vi "E2_Master.vi"() -> ()   [LabVIEW 2020]
uses:
  <vilib>/Instr/_visa.llb/VISA Configure Serial Port (Instr).vi
panel:
  out "Error":errorcluster
  in  "Log":bool
  in  "UpdateTime":bool
  in  "ClearShutdown":bool
  in  "ClearWakeup":bool
  in  "Custom String":string
  in  "SendCustom":bool
  in  "ClearErrors":bool
  in  "Set Shutdown":bool
  in  "Shutdown Time":timestamp
  in  "Wakeup Time":timestamp
  in  "Set Wakeup":bool
  in  "Stop":bool
  in  "Start":bool
  in  "Write Buffer":string
  out "Laser":string
  out "Pump":string
  in  "Disconnect":bool
  in  "Initialize":bool
  in  "VISA Resource Name":refnum<visa-resource-name>
  in  "Resource Name":refnum<visa-resource-name>="Element2"
  in  "Status":bool
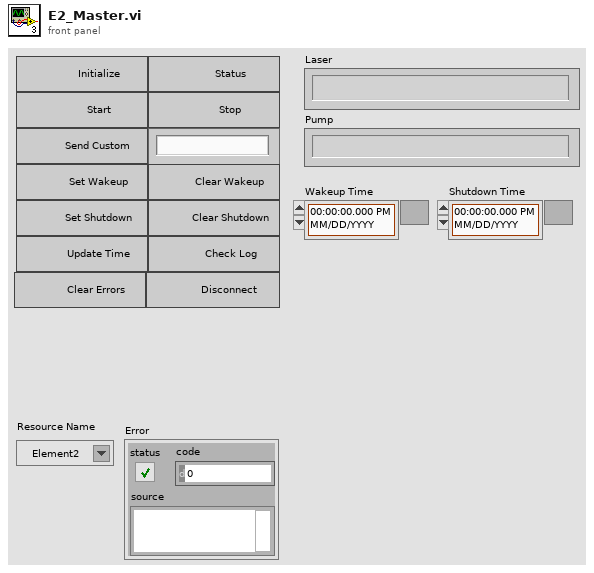
[diagram p1: front panel]
types:
  T1 = enum32{"Invalid", "Standard", "Closed", "Hidden", "Minimized", "Maximized"}
  T2 = enum32{"invalid app kind", "Development System", "Run Time System", "Student Edition", "Embedded LabVIEW", "Evaluation", "Custom"}
  T3 = enum16{"open", "replace", "create", "open or create", "replace or create", "replace or create with confirmation"}
  T4 = cluster{"Core":cluster{"Current VI Reference":refnum<vi>, "Close Panel on Exit?":bool}, "Your Boolean data":bool, "Your string data":string, "VISA Resource Name":refnum<visa-resource-name>, "Write Buffer":string, "Laser Status":string, "Pump Status":string}
  T5 = cluster{"Current VI Reference":refnum<vi>, "Close Panel on Exit?":bool}
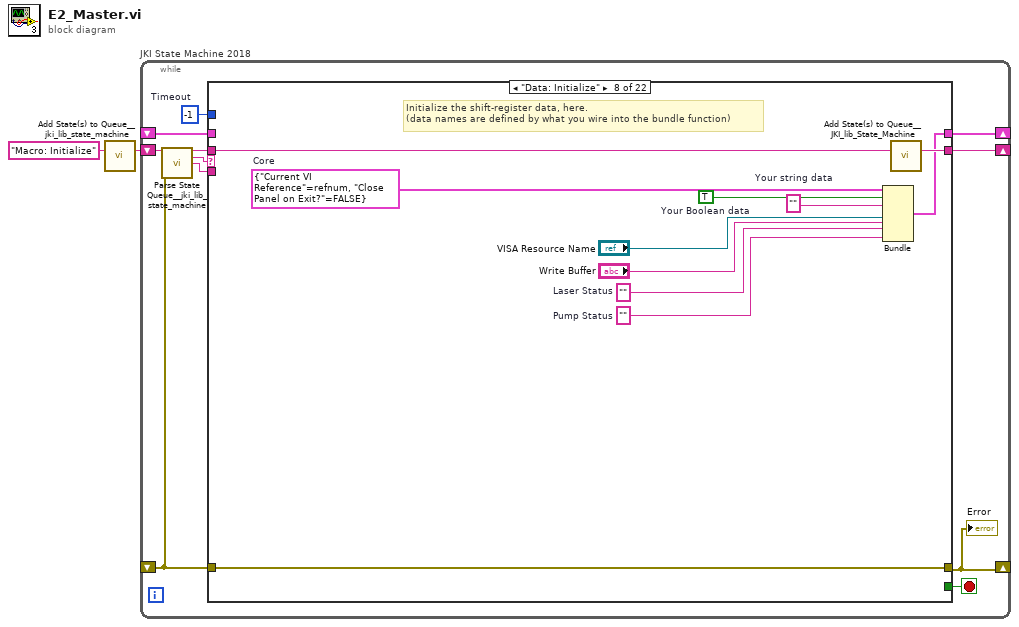
[diagram p0: block diagram]
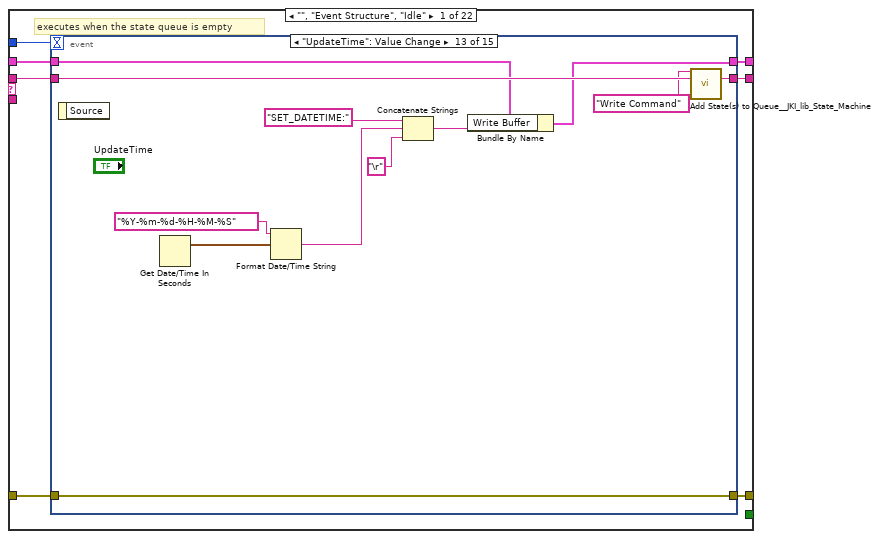
[diagram p2: hidden frame]
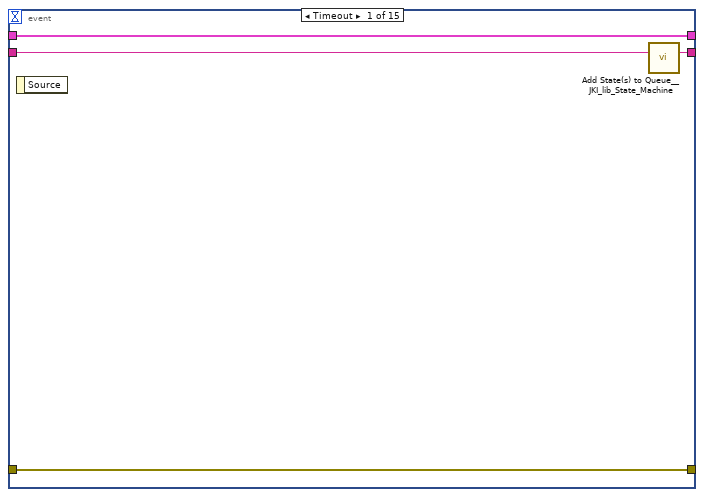
[diagram p3: hidden frame]
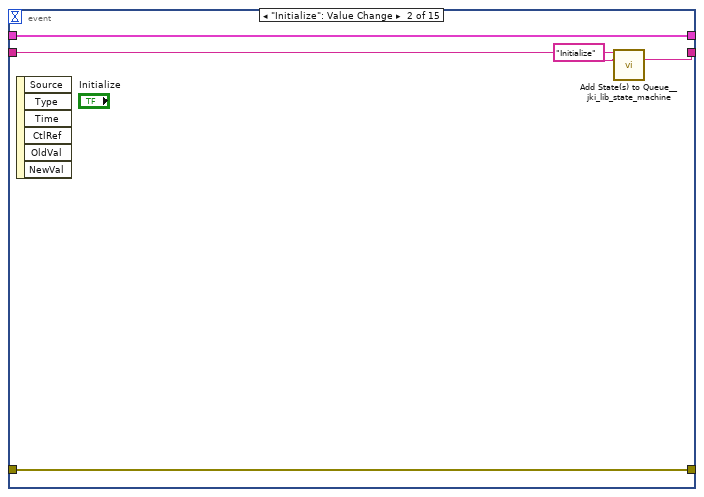
[diagram p4: hidden frame]
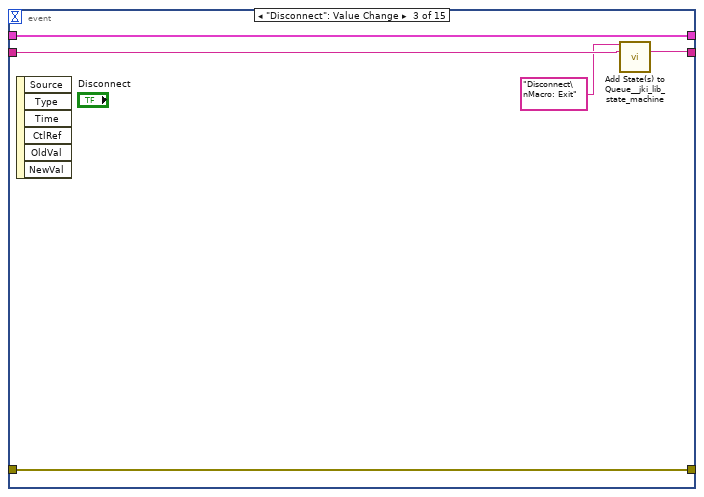
[diagram p5: hidden frame]
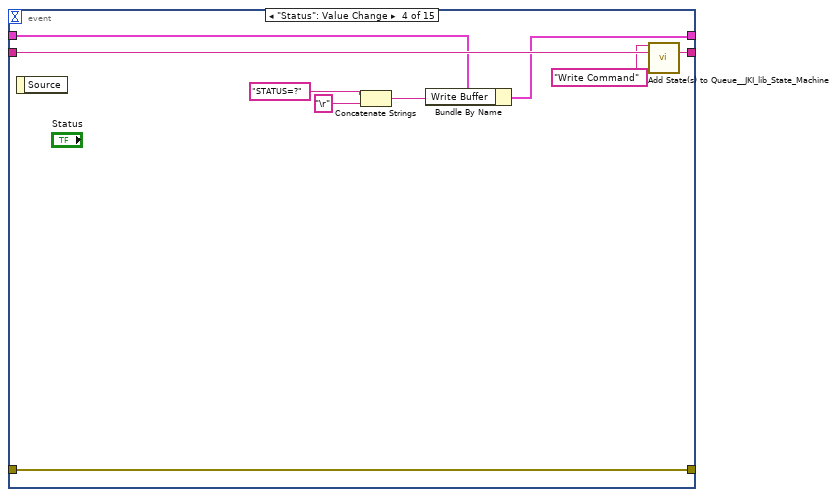
[diagram p6: hidden frame]
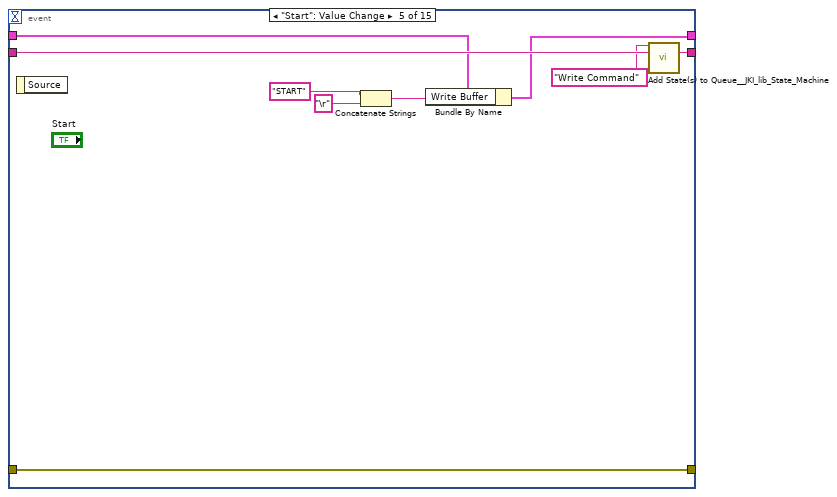
[diagram p7: hidden frame]
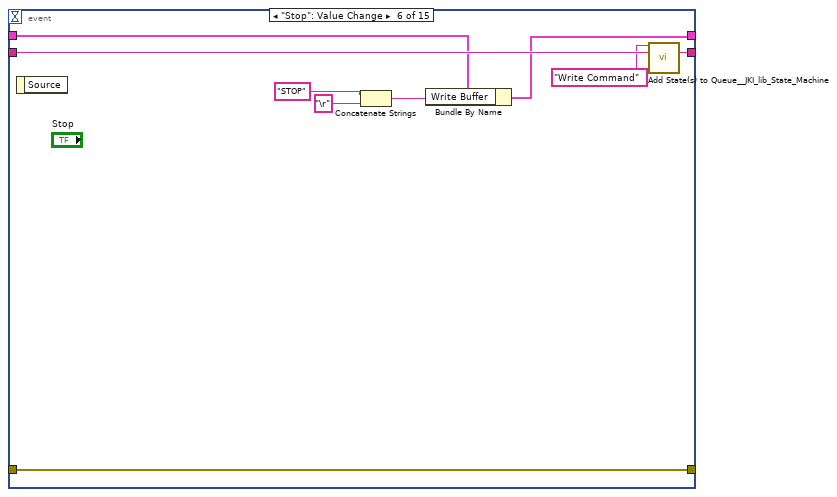
[diagram p8: hidden frame]
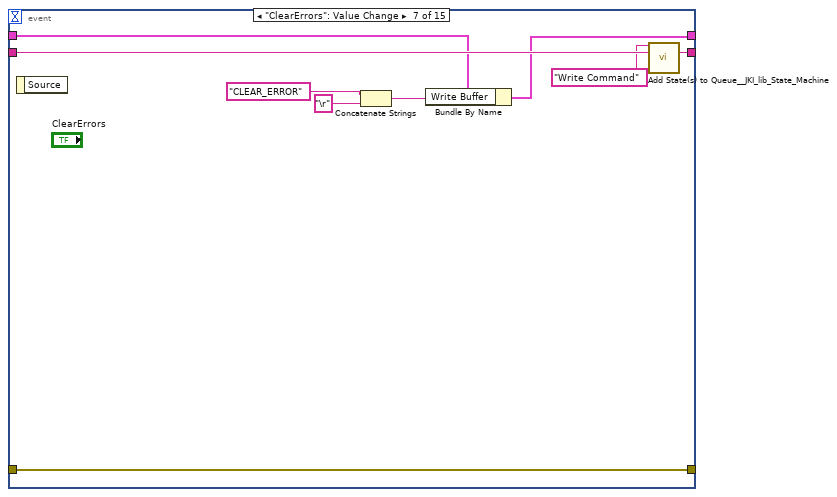
[diagram p9: hidden frame]
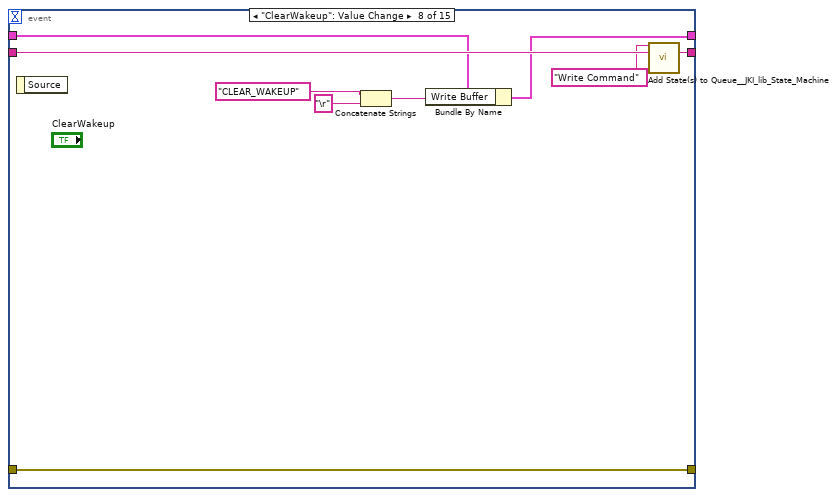
[diagram p10: hidden frame]
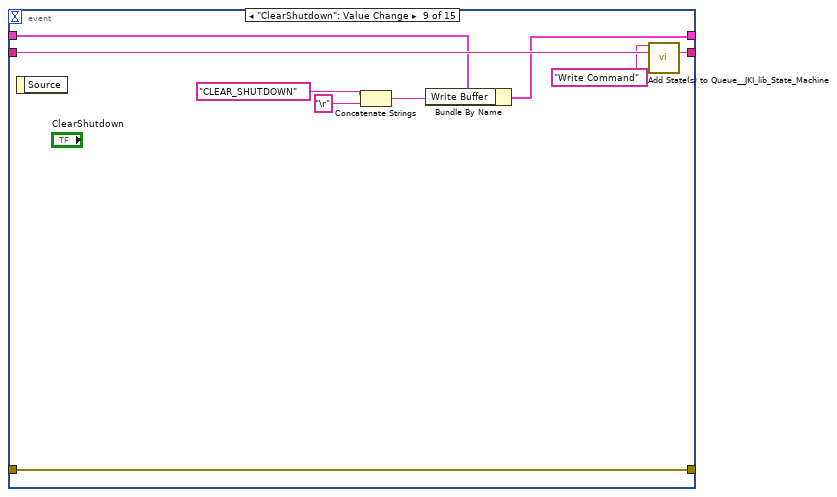
[diagram p11: hidden frame]
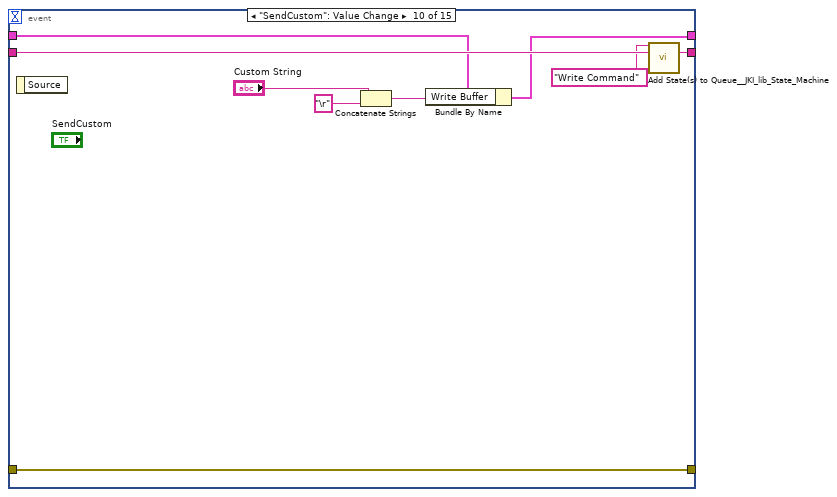
[diagram p12: hidden frame]
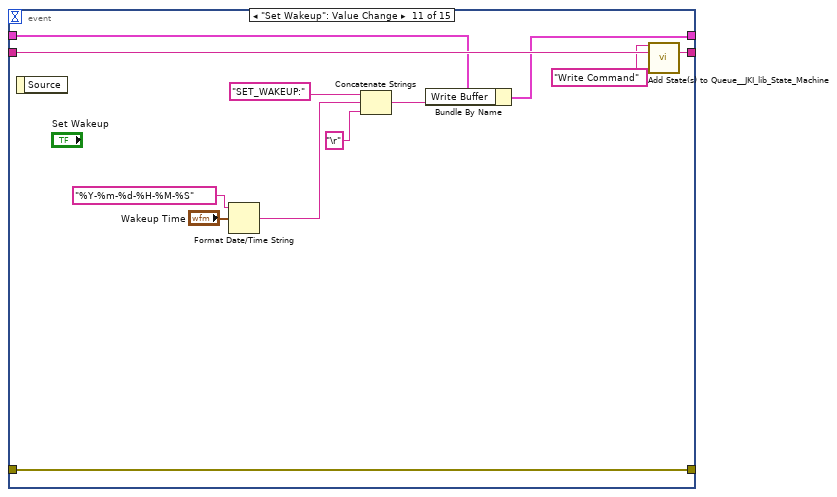
[diagram p13: hidden frame]
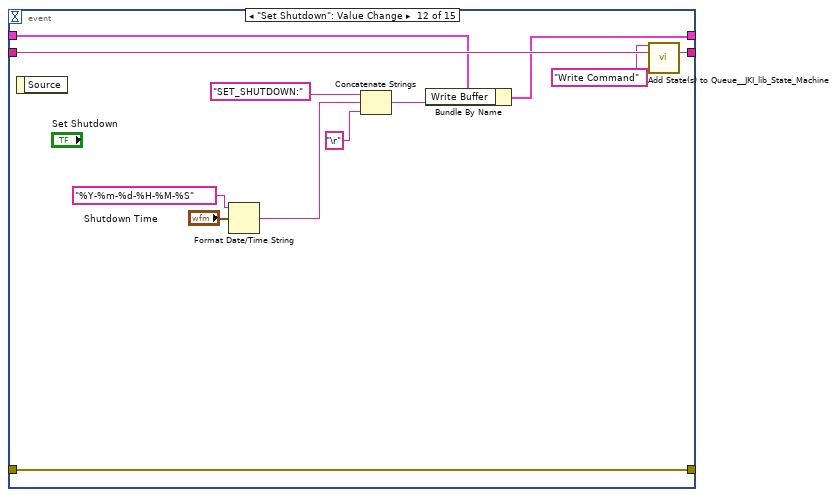
[diagram p14: hidden frame]
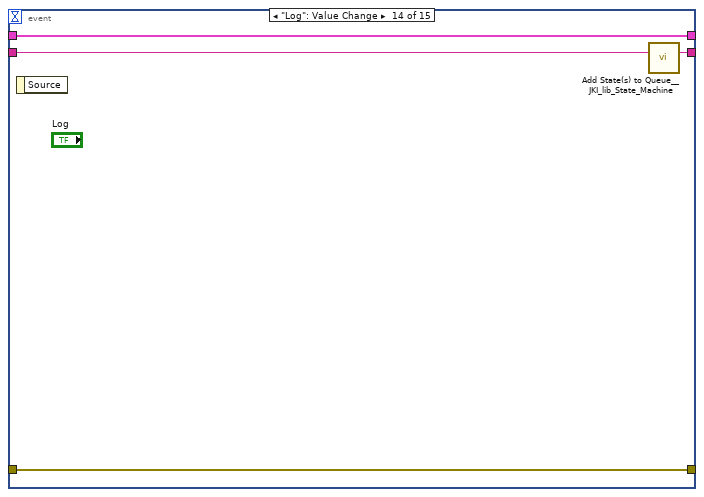
[diagram p15: hidden frame]
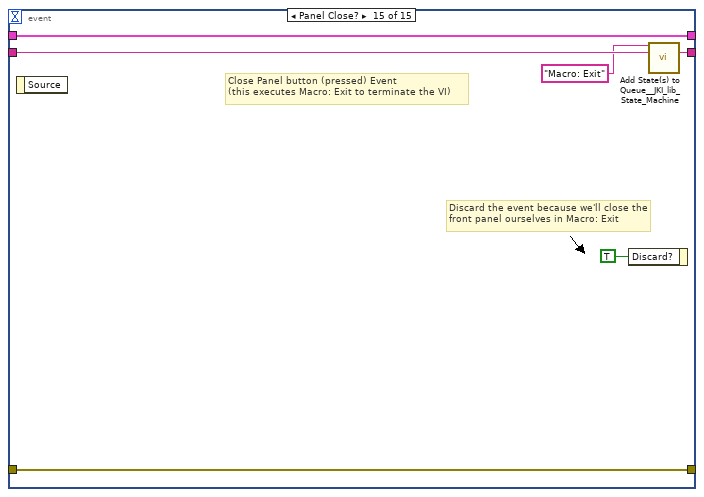
[diagram p16: hidden frame]
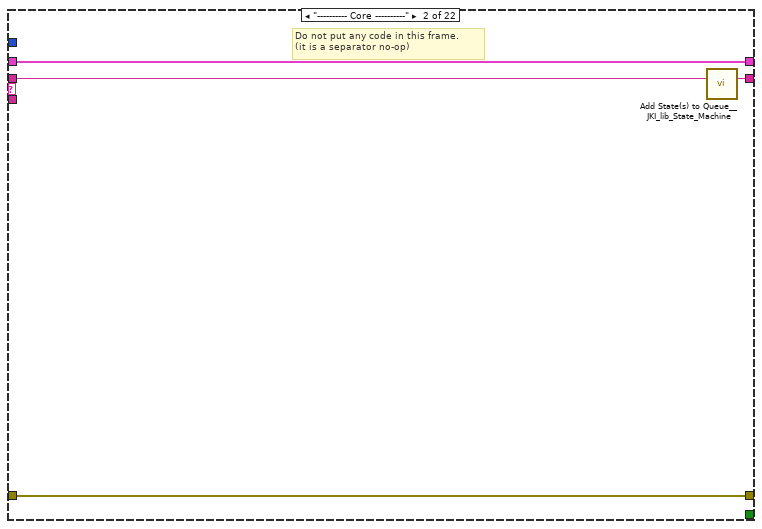
[diagram p17: hidden frame]
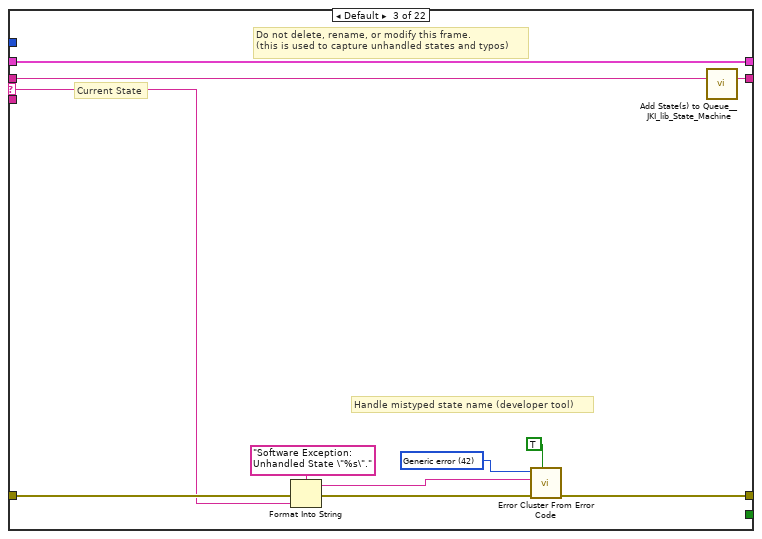
[diagram p18: hidden frame]
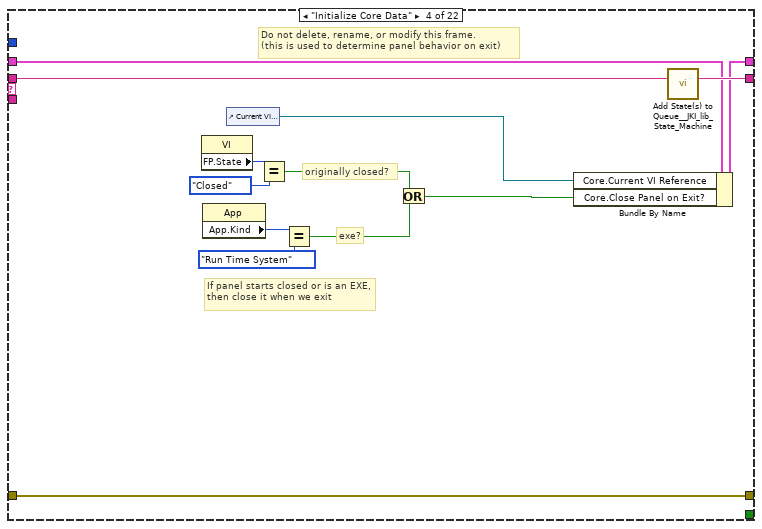
[diagram p19: hidden frame]
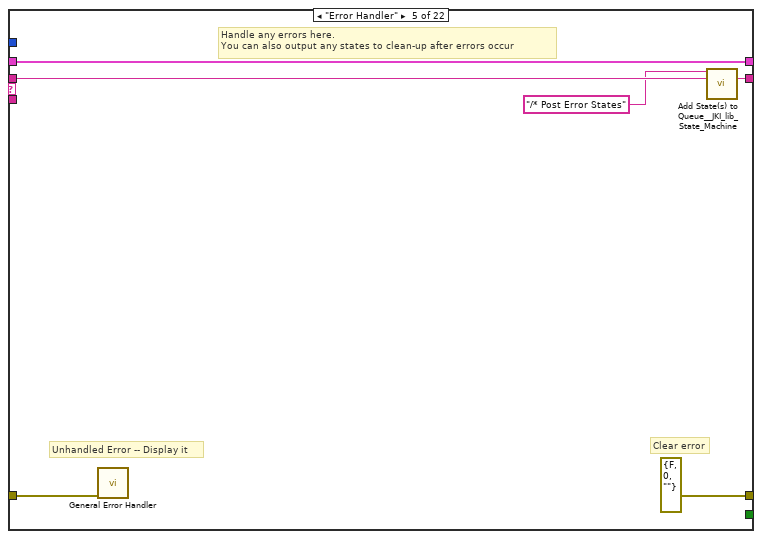
[diagram p20: hidden frame]
diagram:
  n1 = call <vilib>:"Add State(s) to Queue__jki_lib_state_machine.vi"("State(s) in (\"\")"="Macro: Initialize") -> ("States Out"=w2:string)  [unwired: 14 in]
  n2 = while "JKI State Machine 2018" {
    shift-right: [w6] -> _
    shift-left: _ -> [w5]
    shift-right: [w9] -> _
    shift-left: _ -> [w3]
    shift-right: [w8] -> _
    shift-left: w2 -> [w10]
    stop <- w7 stop-if-true
    w4 = -1  # Timeout
    n3 = call <vilib>:"Parse State Queue__jki_lib_state_machine.vi"("State Queue"=w10, "Error In (no error)"=w3) -> ("Remaining States"=w12:string, "Current State"=w13:string, "Arguments"=w11:string)  [unwired: 11 in]
    n4 = case shown="\"Data: Initialize\"" w13 {
      selector: w13 -> [_ _ w148 _ _ _ _ _ _ _ _ _ _ _ _ _ _ _ _ _ _ _]
      tunnel: w12 -> [w20 w147 w152 w171 w177 w182 w186 w197 w203 w207 w211 w217 w228 w297 w302 w312 w316 w330 w338 w360 w383 w411]
      tunnel: w11 -> [_ _ _ _ _ _ _ _ _ _ _ w212 w222 _ _ _ _ _ _ _ _ _]
      tunnel: w5 -> [w18 w144 w150 w164 w174 w180 w183 _ w198 w204 w209 w215 w224 w294 w299 w309 w313 w322 w332 w342 w381 w407]
      tunnel: [w17 w145 w154 w168 errorcluster {"status"=FALSE, "code"=0, "source"=""} ("error out") w179 w184 w194 w199 w205 w208 w213 w225 w295 w300 w310 w314 w318 w334 w346 w374 w397] -> w9
      tunnel: w3 -> [w16 w145 w153 w168 w173 w179 w184 w194 w200 w205 w208 w214 w226 w295 w300 w310 w314 w319 w333 w352 w379 w398]
      tunnel: [w19 w146 w151 w170 w176 w181 w185 w196 w202 w206 w210 w216 w227 w296 w301 w311 w315 w329 w337 w359 w382 w410] -> w8
      tunnel: [_ _ _ _ _ TRUE _ _ _ _ _ _ _ _ _ _ _ _ _ _ _ _] -> w7
      tunnel: [w15 w144 w150 w169 w174 w180 w183 w195 w198 w204 w209 w215 w224 w294 w299 w309 w313 w321 w332 w341 w381 w407] -> w6
      tunnel: w4 -> [w14 _ _ _ _ _ _ _ _ _ _ _ _ _ _ _ _ _ _ _ _ _]
      frame "", "Event Structure", "Idle" {
        # "executes when the state queue is empty"
        n5 = event shown="[12] \"UpdateTime\": Value Change" {
          selector: _ -> [_ _ _ _ _ _ _ _ _ _ _ _ _ _ _]
          dyn-events: _ -> [_ _ _ _ _ _ _ _ _ _ _ _ _ _ _]
          timeout: w14 -> [_ _ _ _ _ _ _ _ _ _ _ _ _ _ _]
          tunnel: w20 -> [w24 w27 w32 w43 w52 w61 w70 w79 w88 w97 w109 w121 w133 w137 w143]
          tunnel: [w23 w28 w33 w42 w51 w60 w69 w78 w87 w96 w108 w120 w132 w136 w142] -> w19
          tunnel: w18 -> [w21 w29 w34 w39 w48 w57 w66 w75 w84 w93 w105 w117 w129 w134 w140]
          tunnel: [w22 w25 w30 w41 w50 w59 w68 w77 w86 w95 w107 w119 w131 w135 w141] -> w17
          tunnel: w16 -> [w22 w25 w30 w41 w50 w59 w68 w77 w86 w95 w107 w119 w131 w135 w141]
          tunnel: [w21 w29 w34 w38 w47 w56 w65 w74 w83 w92 w104 w116 w128 w134 w140] -> w15
          event Timeout {
            n6 = event-data() -> ()  [unwired: 1 in, 1 out]
            n7 = call <vilib>:"Add State(s) to Queue__JKI_lib_State_Machine.vi"("State(s) in (\"\")"=w24) -> ("States Out"=w23:string)  [unwired: 14 in]
          }
          event "Initialize": Value Change {
            n8 = event-data() -> ()  [unwired: 1 in, 6 out]
            n9 = call <vilib>:"Add State(s) to Queue__jki_lib_state_machine.vi"("State(s) in Front (\"\")"="Initialize" ("State(s) in Front (\"\")"), "State(s) in (\"\")"=w27) -> ("States Out"=w28:string)  [unwired: 13 in]
          }
          event "Disconnect": Value Change {
            n10 = event-data() -> ()  [unwired: 1 in, 6 out]
            n11 = call <vilib>:"Add State(s) to Queue__jki_lib_state_machine.vi"("State(s) in Front (\"\")"="Disconnect\nMacro: Exit" ("State(s) in Front (\"\")"), "State(s) in (\"\")"=w32) -> ("States Out"=w33:string)  [unwired: 13 in]
          }
          event "Status": Value Change {
            n12 = event-data() -> ()  [unwired: 1 in, 1 out]
            n13 = Concatenate Strings("STATUS=?" ("string"), "\r" ("string")) -> (w35:string)
            n14 = Bundle By Name(cluster=w39, "Write Buffer"=w35) -> (w38:T4)
            n15 = call <vilib>:"Add State(s) to Queue__JKI_lib_State_Machine.vi"("State(s) in Front (\"\")"="Write Command", "State(s) in (\"\")"=w43) -> ("States Out"=w42:string)  [unwired: 13 in]
          }
          event "Start": Value Change {
            n16 = event-data() -> ()  [unwired: 1 in, 1 out]
            n17 = Concatenate Strings("START" ("string"), "\r" ("string")) -> (w44:string)
            n18 = Bundle By Name(cluster=w48, "Write Buffer"=w44) -> (w47:T4)
            n19 = call <vilib>:"Add State(s) to Queue__JKI_lib_State_Machine.vi"("State(s) in Front (\"\")"="Write Command", "State(s) in (\"\")"=w52) -> ("States Out"=w51:string)  [unwired: 13 in]
          }
          event "Stop": Value Change {
            n20 = event-data() -> ()  [unwired: 1 in, 1 out]
            n21 = Concatenate Strings("STOP" ("string"), "\r" ("string")) -> (w53:string)
            n22 = Bundle By Name(cluster=w57, "Write Buffer"=w53) -> (w56:T4)
            n23 = call <vilib>:"Add State(s) to Queue__JKI_lib_State_Machine.vi"("State(s) in Front (\"\")"="Write Command", "State(s) in (\"\")"=w61) -> ("States Out"=w60:string)  [unwired: 13 in]
          }
          event "ClearErrors": Value Change {
            n24 = event-data() -> ()  [unwired: 1 in, 1 out]
            n25 = Concatenate Strings("CLEAR_ERROR" ("string"), "\r" ("string")) -> (w62:string)
            n26 = Bundle By Name(cluster=w66, "Write Buffer"=w62) -> (w65:T4)
            n27 = call <vilib>:"Add State(s) to Queue__JKI_lib_State_Machine.vi"("State(s) in Front (\"\")"="Write Command", "State(s) in (\"\")"=w70) -> ("States Out"=w69:string)  [unwired: 13 in]
          }
          event "ClearWakeup": Value Change {
            n28 = event-data() -> ()  [unwired: 1 in, 1 out]
            n29 = Concatenate Strings("CLEAR_WAKEUP" ("string"), "\r" ("string")) -> (w71:string)
            n30 = Bundle By Name(cluster=w75, "Write Buffer"=w71) -> (w74:T4)
            n31 = call <vilib>:"Add State(s) to Queue__JKI_lib_State_Machine.vi"("State(s) in Front (\"\")"="Write Command", "State(s) in (\"\")"=w79) -> ("States Out"=w78:string)  [unwired: 13 in]
          }
          event "ClearShutdown": Value Change {
            n32 = event-data() -> ()  [unwired: 1 in, 1 out]
            n33 = Concatenate Strings("CLEAR_SHUTDOWN" ("string"), "\r" ("string")) -> (w80:string)
            n34 = Bundle By Name(cluster=w84, "Write Buffer"=w80) -> (w83:T4)
            n35 = call <vilib>:"Add State(s) to Queue__JKI_lib_State_Machine.vi"("State(s) in Front (\"\")"="Write Command", "State(s) in (\"\")"=w88) -> ("States Out"=w87:string)  [unwired: 13 in]
          }
          event "SendCustom": Value Change {
            n36 = event-data() -> ()  [unwired: 1 in, 1 out]
            n37 = Concatenate Strings("Custom String", "\r" ("string")) -> (w90:string)
            n38 = Bundle By Name(cluster=w93, "Write Buffer"=w90) -> (w92:T4)
            n39 = call <vilib>:"Add State(s) to Queue__JKI_lib_State_Machine.vi"("State(s) in Front (\"\")"="Write Command", "State(s) in (\"\")"=w97) -> ("States Out"=w96:string)  [unwired: 13 in]
          }
          event "Set Wakeup": Value Change {
            n40 = event-data() -> ()  [unwired: 1 in, 1 out]
            n41 = Format Date/Time String(time format string (%c)="%Y-%m-%d-%H-%M-%S", seconds (now)="Wakeup Time") -> (date/time string=w98:string)  [unwired: 1 in]
            n42 = Concatenate Strings("SET_WAKEUP:" ("string"), w98, "\r" ("string")) -> (w102:string)
            n43 = Bundle By Name(cluster=w105, "Write Buffer"=w102) -> (w104:T4)
            n44 = call <vilib>:"Add State(s) to Queue__JKI_lib_State_Machine.vi"("State(s) in Front (\"\")"="Write Command", "State(s) in (\"\")"=w109) -> ("States Out"=w108:string)  [unwired: 13 in]
          }
          event "Set Shutdown": Value Change {
            n45 = event-data() -> ()  [unwired: 1 in, 1 out]
            n46 = Format Date/Time String(time format string (%c)="%Y-%m-%d-%H-%M-%S", seconds (now)="Shutdown Time") -> (date/time string=w110:string)  [unwired: 1 in]
            n47 = Concatenate Strings("SET_SHUTDOWN:" ("string"), w110, "\r" ("string")) -> (w114:string)
            n48 = Bundle By Name(cluster=w117, "Write Buffer"=w114) -> (w116:T4)
            n49 = call <vilib>:"Add State(s) to Queue__JKI_lib_State_Machine.vi"("State(s) in Front (\"\")"="Write Command", "State(s) in (\"\")"=w121) -> ("States Out"=w120:string)  [unwired: 13 in]
          }
          event "UpdateTime": Value Change {
            n50 = event-data() -> ()  [unwired: 1 in, 1 out]
            n51 = Get Date/Time In Seconds() -> (seconds since 1Jan1904=w122:timestamp)
            n52 = Format Date/Time String(time format string (%c)="%Y-%m-%d-%H-%M-%S", seconds (now)=w122) -> (date/time string=w123:string)  [unwired: 1 in]
            n53 = Concatenate Strings("SET_DATETIME:" ("string"), w123, "\r" ("string")) -> (w126:string)
            n54 = Bundle By Name(cluster=w129, "Write Buffer"=w126) -> (w128:T4)
            n55 = call <vilib>:"Add State(s) to Queue__JKI_lib_State_Machine.vi"("State(s) in Front (\"\")"="Write Command", "State(s) in (\"\")"=w133) -> ("States Out"=w132:string)  [unwired: 13 in]
          }
          event "Log": Value Change {
            n56 = event-data() -> ()  [unwired: 1 in, 1 out]
            n57 = call <vilib>:"Add State(s) to Queue__JKI_lib_State_Machine.vi"("State(s) in (\"\")"=w137) -> ("States Out"=w136:string)  [unwired: 14 in]
          }
          event Panel Close? {
            # "Discard the event because we'll close the front panel ourselves in Macro: Exit"
            # "Close Panel button (pressed) Event\n(this executes Macro: Exit to terminate the VI)"
            n58 = event-data() -> ()  [unwired: 1 in, 1 out]
            n59 = event-data("Discard?"=TRUE) -> ()  [unwired: 1 in, 1 out]
            n60 = call <vilib>:"Add State(s) to Queue__JKI_lib_State_Machine.vi"("State(s) in Front (\"\")"="Macro: Exit", "State(s) in (\"\")"=w143) -> ("States Out"=w142:string)  [unwired: 13 in]
          }
        }
      }
      frame "---------- Core ----------" {
        # "Do not put any code in this frame.\n(it is a separator no-op)"
        n61 = call <vilib>:"Add State(s) to Queue__JKI_lib_State_Machine.vi"("State(s) in (\"\")"=w147) -> ("States Out"=w146:string)  [unwired: 14 in]
      }
      frame Default {
        w157 = 42 items=["No error", "Argument error", "Memory is full", "Out of zone", "End of file", "File already open", "Generic file I/O error", "File not found", "File permission error", "Disk is full", "Duplicate path", "Too many files open", "System feature not enabled", "Resource file not found", "Cannot add resource", "Resource not found", "Image not found", "Image memory error", "Pen does not exist", "Config type invalid", "Config token not found", "Config parse error", "Config memory error", "Bad external code format", "Bad external code offset", "External code not present", "Null window", "Destroy window error", "Null menu", "Print aborted", "Bad print record", "Print driver error", "Windows error during printing", "Memory error during printing", "Print dialog error", "Generic print error", "Invalid device refnum", "Device not found", "Device parameter error", "Device unit error", "Cannot open device", "Device call aborted", "Generic error", "Cancelled by user", "Object ID too low", "Object ID too high", "Object not in heap", "Unknown heap", "Unknown object (invalid DefProc)", "Unknown object (DefProc not in table)", "Message out of range", "Invalid (null) method", "Unknown message", "Manager call not supported", "Bad address", "Network operation in progress", "Network operation timed out", "Connection is busy", "Network attribute not supported", "Network error", "Address in use", "System out of memory", "Connection aborted", "Connection refused", "Not connected", "Already connected", "Connection closed", "Initialization error (interapplication manager)", "Bad occurrence", "Wait on unbound occurrence handler", "Occurrence queue overflow", "Datalog type conflict", "Unused", "Unrecognized type (interapplication manager)", "Memory corrupt", "Failed to make temporary DLL", "Old CIN version", "Drag socket not found", "Failed to load drop-object", "Failed to register OLE object", "Failed to release OLE object", "Format specifier type mismatch", "Unknown format specifier", "Too few format specifiers", "Too many format specifiers", "Scan failed", "Newer CIN version", "Error converting to variant", "Runtime menu error", "Password tampered", "Variant attribute not found", "Incompatible variant data type", "Event data is not available", "Event Store is not present", "Occurrence is not found", "Event Queue is not created", "Event info is not available", "Refnum passed is NULL", "Error retrieving Class GUID", "Error retrieving CoClass GUID", "Error retrieving TypeLib GUID.", "Bad built application magic bytes.", "Specific driver is different from the specific driver associated with the Logical Name.", "There is no session opened to the class driver.", "Max Error", "MAX - Error with config objects", "MAX - Error loading configuration", "MAX - Group not supported"]
        # "Current State"
        # "Do not delete, rename, or modify this frame.\n(this is used to capture unhandled states and typos)"
        # "Handle mistyped state name (developer tool)"
        n62 = Format Into String(format string="Software Exception: Unhandled State \"%s\"." ("message"), error in=w153, w148) -> (resulting string=w156:string, error out=w155:errorcluster)  [unwired: 1 in]
        n63 = call <vilib>:"Error Cluster From Error Code.vi"("show call chain? (False)"=TRUE, "error in (no error)"=w155, "error message (\"\")"=w156, "error code (0)"=w157) -> ("error out"=w154:errorcluster)  [unwired: 5 in]
        n64 = call <vilib>:"Add State(s) to Queue__JKI_lib_State_Machine.vi"("State(s) in (\"\")"=w152) -> ("States Out"=w151:string)  [unwired: 14 in]
      }
      frame "Initialize Core Data" {
        # "Do not delete, rename, or modify this frame.\n(this is used to determine panel behavior on exit)"
        # "originally closed?"
        # "exe?"
        # "If panel starts closed or is an EXE, then close it when we exit"
        n65 = property class="VI"() -> ("FP.State"=w161:T1)  [unwired: 2 in, 2 out]
        n66 = property class="App"() -> ("App.Kind"=w167:T2)  [unwired: 2 in, 2 out]
        n67 = control-ref of="Current VI Reference"() -> (w162:refnum<vi>)
        n68 = Equal?(x=w161, y=T1."Closed" ("Front Panel Window:State")) -> (x = y?=w159:bool)
        n69 = Equal?(x=w167, y=T2."Run Time System" ("Application:Kind")) -> (x = y?=w165:bool)
        n70 = Or(x=w159, y=w165) -> (x .or. y?=w163:bool)
        n71 = Bundle By Name(cluster=w164, "Core.Current VI Reference"=w162, "Core.Close Panel on Exit?"=w163) -> (w169:T4)
        n72 = call <vilib>:"Add State(s) to Queue__JKI_lib_State_Machine.vi"("State(s) in (\"\")"=w171) -> ("States Out"=w170:string)  [unwired: 14 in]
      }
      frame "Error Handler" {
        # "Unhandled Error -- Display it"
        # "Handle any errors here.\nYou can also output any states to clean-up after errors occur"
        # "Clear error"
        n73 = call <vilib>:"General Error Handler.vi"("error in (no error)"=w173) -> ()  [unwired: 10 in, 5 out]
        n74 = call <vilib>:"Add State(s) to Queue__JKI_lib_State_Machine.vi"("State(s) in Front (\"\")"="/* Post Error States", "State(s) in (\"\")"=w177) -> ("States Out"=w176:string)  [unwired: 13 in]
      }
      frame "Exit" {
        # "Do not put any code in this frame.\n(No errors that occur here will be handled.)"
        n75 = call <vilib>:"Add State(s) to Queue__JKI_lib_State_Machine.vi"("State(s) in (\"\")"=w182) -> ("States Out"=w181:string)  [unwired: 14 in]
      }
      frame "---------- Data ----------" {
        # "Do not put any code in this frame.\n(It is a separator no-op. You can make a copy of this frame to create a new Data frame)"
        n76 = call <vilib>:"Add State(s) to Queue__JKI_lib_State_Machine.vi"("State(s) in (\"\")"=w186) -> ("States Out"=w185:string)  [unwired: 14 in]
      }
      frame "Data: Initialize" {
        w187 = ""  # Pump Status
        w188 = ""  # Laser Status
        w191 = T5 {"Current VI Reference"=refnum, "Close Panel on Exit?"=FALSE}  # Core
        w193 = TRUE  # Your Boolean data
        w192 = ""  # Your string data
        # "Initialize the shift-register data, here.\n(data names are defined by what you wire into the bundle function)"
        n77 = Bundle("Core"=w191, "Your Boolean data"=w193, "Your string data"=w192, "VISA Resource Name"="VISA Resource Name", "Write Buffer"="Write Buffer", "Laser Status"=w188, "Pump Status"=w187) -> (w195:T4)  [unwired: 1 in]
        n78 = call <vilib>:"Add State(s) to Queue__JKI_lib_State_Machine.vi"("State(s) in (\"\")"=w197) -> ("States Out"=w196:string)  [unwired: 14 in]
      }
      frame "Data: Cleanup" {
        # "Cleanup any data and references, here.\n(this is called automatically, by the Macro: Exit)"
        n79 = Unbundle By Name(w198) -> ("Core.Current VI Reference"=w201:refnum<vi>)
        n80 = Close Reference(reference=w201, error in (no error)=w200) -> (error out=w199:errorcluster)
        n81 = call <vilib>:"Add State(s) to Queue__JKI_lib_State_Machine.vi"("State(s) in (\"\")"=w203) -> ("States Out"=w202:string)  [unwired: 14 in]
      }
      frame "---------- UI ----------" {
        # "Do not put any code in this frame.\n(It is a separator no-op. You can make a copy of this frame to create a new UI frame)"
        n82 = call <vilib>:"Add State(s) to Queue__JKI_lib_State_Machine.vi"("State(s) in (\"\")"=w207) -> ("States Out"=w206:string)  [unwired: 14 in]
      }
      frame "UI: Initialize" {
        # "Initialize the User Interface, here.\n(this is called automatically, by the Macro: Init)"
        n83 = call <vilib>:"Add State(s) to Queue__JKI_lib_State_Machine.vi"("State(s) in (\"\")"=w211) -> ("States Out"=w210:string)  [unwired: 14 in]
      }
      frame "UI: Cursor Set" {
        # "Argument"
        # "Set and Unset Cursor Busy.\n(Usage: \"UI: Cursor Set >> Busy|Idle\")"
        n84 = case shown="\"Idle\", Default" w212 {
          tunnel: w214 -> [w219 w221]
          tunnel: [w218 w220] -> w213
          frame "Idle", Default {
            n85 = call <vilib>:"Unset Busy.vi"("error in (no error)"=w219) -> ("error out"=w218:errorcluster)  [unwired: 10 in]
          }
          frame "Busy" {
            n86 = call <vilib>:"Set Busy.vi"("error in (no error)"=w221) -> ("error out"=w220:errorcluster)  [unwired: 9 in, 1 out]
          }
        }
        n87 = call <vilib>:"Add State(s) to Queue__JKI_lib_State_Machine.vi"("State(s) in (\"\")"=w217) -> ("States Out"=w216:string)  [unwired: 14 in]
      }
      frame "UI: Front Panel State" {
        # "Argument"
        # "Set Front Panel Open or Closed\n(Usage: \"UI: Front Panel State >> Open|Close\")"
        n88 = Unbundle By Name(w224) -> ("Core.Current VI Reference"=w223:refnum<vi>)
        n89 = case shown="\"Minimize\", \"Minimized\"" w222 {
          tunnel: w226 -> [w234 w249 w260 w273 w286]
          tunnel: [w236 w250 w262 w275 w288] -> w225
          tunnel: w223 -> [w235 w247 w261 w274 w287]
          frame "Open", "Standard", Default {
            w229 = T1."Standard" ("State")
            n90 = property class="VI"(reference=w235, error in=w234) -> (reference out=w232:refnum<vi>, error out=w233:errorcluster, "FP.State"=w231:T1)
            n91 = Not Equal?(x=w231, y=w229) -> (x != y?=w230:bool)
            n92 = case shown="True" w230 {
              tunnel: [w240 w242] -> w236
              tunnel: w233 -> [w239 w242]
              tunnel: w232 -> [w238 _]
              tunnel: w229 -> [w237 _]
              frame True {
                n93 = invoke class="VI" method="FP.Open"(reference=w238, error in=w239, "Activate"=TRUE, "State"=w237) -> (error out=w240:errorcluster)  [unwired: 1 in, 4 out]
              }
              frame False {
              }
            }
          }
          frame "Close", "Closed" {
            n94 = property class="VI"(reference=w247, error in=w249) -> (reference out=w246:refnum<vi>, error out=w248:errorcluster, "FP.State"=w244:T1)
            n95 = Not Equal?(x=w244, y=T1."Closed" ("Front Panel Window:State")) -> (x != y?=w243:bool)
            n96 = case shown="True" w243 {
              tunnel: [w251 w254] -> w250
              tunnel: w248 -> [w251 w253]
              tunnel: w246 -> [_ w252]
              frame False {
              }
              frame True {
                n97 = invoke class="VI" method="FP.Close"(reference=w252, error in=w253) -> (error out=w254:errorcluster)  [unwired: 1 in, 2 out]
              }
            }
          }
          frame "Hidden", "Hide" {
            w255 = T1."Hidden" ("State")
            n98 = property class="VI"(reference=w261, error in=w260) -> (reference out=w258:refnum<vi>, error out=w259:errorcluster, "FP.State"=w257:T1)
            n99 = Not Equal?(x=w257, y=w255) -> (x != y?=w256:bool)
            n100 = case shown="True" w256 {
              tunnel: [w266 w267] -> w262
              tunnel: w259 -> [w265 w267]
              tunnel: w258 -> [w264 _]
              tunnel: w255 -> [w263 _]
              frame True {
                n101 = invoke class="VI" method="FP.Open"(reference=w264, error in=w265, "State"=w263) -> (error out=w266:errorcluster)  [unwired: 2 in, 4 out]
              }
              frame False {
              }
            }
          }
          frame "Minimize", "Minimized" {
            w268 = T1."Minimized" ("State")
            n102 = property class="VI"(reference=w274, error in=w273) -> (reference out=w271:refnum<vi>, error out=w272:errorcluster, "FP.State"=w270:T1)
            n103 = Not Equal?(x=w270, y=w268) -> (x != y?=w269:bool)
            n104 = case shown="True" w269 {
              tunnel: [w279 w280] -> w275
              tunnel: w272 -> [w278 w280]
              tunnel: w271 -> [w277 _]
              tunnel: w268 -> [w276 _]
              frame True {
                n105 = invoke class="VI" method="FP.Open"(reference=w277, error in=w278, "State"=w276) -> (error out=w279:errorcluster)  [unwired: 2 in, 4 out]
              }
              frame False {
              }
            }
          }
          frame "Maximize", "Maximized" {
            w281 = T1."Maximized" ("State")
            n106 = property class="VI"(reference=w287, error in=w286) -> (reference out=w284:refnum<vi>, error out=w285:errorcluster, "FP.State"=w283:T1)
            n107 = Not Equal?(x=w283, y=w281) -> (x != y?=w282:bool)
            n108 = case shown="True" w282 {
              tunnel: [w292 w293] -> w288
              tunnel: w285 -> [w291 w293]
              tunnel: w284 -> [w290 _]
              tunnel: w281 -> [w289 _]
              frame True {
                n109 = invoke class="VI" method="FP.Open"(reference=w290, error in=w291, "State"=w289) -> (error out=w292:errorcluster)  [unwired: 2 in, 4 out]
              }
              frame False {
              }
            }
          }
        }
        n110 = call <vilib>:"Add State(s) to Queue__JKI_lib_State_Machine.vi"("State(s) in (\"\")"=w228) -> ("States Out"=w227:string)  [unwired: 14 in]
      }
      frame "---------- Macro ----------" {
        # "Do not put any code in this frame.\n(It is a separator no-op. You can make a copy of this frame to create a new Macro frame)"
        n111 = call <vilib>:"Add State(s) to Queue__JKI_lib_State_Machine.vi"("State(s) in (\"\")"=w297) -> ("States Out"=w296:string)  [unwired: 14 in]
      }
      frame "Macro: Initialize" {
        w298 = "Data: Initialize\nInitialize Core Data\nUI: Initialize\nUI: Front Panel State >> Open"  # Data: Initialize Initialize Core Data UI: Initialize UI: Front Panel State >> Open
        # "Initialization Macro\n(This is called once, when the VI starts)"
        n112 = call <vilib>:"Add State(s) to Queue__JKI_lib_State_Machine.vi"("State(s) in Front (\"\")"=w298, "State(s) in (\"\")"=w302) -> ("States Out"=w301:string)  [unwired: 13 in]
      }
      frame "Macro: Exit" {
        # "Exit Macro\n(This is called once, when the VI exits)"
        n113 = Unbundle By Name(w309) -> ("Core.Close Panel on Exit?"=w308:bool)
        n114 = Select(t="UI: Front Panel State >> Close", s=w308, f="") -> (s? t:f=w305:string)
        n115 = call <vilib>:"Add State(s) to Queue__JKI_lib_State_Machine.vi"("State(s) in (\"\")"=w305, "State(s) at Back (\"\")"="Data: Cleanup\nExit") -> ("States Out"=w303:string)  [unwired: 13 in]
        n116 = call <vilib>:"Add State(s) to Queue__JKI_lib_State_Machine.vi"("State(s) in Front (\"\")"=w303, "State(s) in (\"\")"=w312) -> ("States Out"=w311:string)  [unwired: 13 in]
      }
      frame "---------- New Category ----------" {
        # "Template Separator\n(You can make a copy of, or modify, this frame)"
        n117 = call <vilib>:"Add State(s) to Queue__JKI_lib_State_Machine.vi"("State(s) in (\"\")"=w316) -> ("States Out"=w315:string)  [unwired: 14 in]
      }
      frame "Initialize" {
        w323 = u16 0 items=["None", "XON/XOFF", "RTS/CTS", "XON/XOFF & RTS/CTS", "DTR/DSR", "XON/XOFF & DTR/DSR"]  # flow control (0:none)
        w324 = u16 8  # data bits (8)
        w325 = u32 115200  # baud rate (9600)
        w326 = enum16{"None", "Odd", "Even", "Mark", "Space"}."None"  # parity (0:none)
        # "Do not put any code in this frame.\n(it is a separator no-op)"
        n118 = call-poly "VISA Configure Serial Port"("VISA resource name"="Resource Name", "timeout (10sec)"=u32 1000, "Enable Termination\nChar (T)"=TRUE ("Enable Termination\nChar (T)"), "baud rate (9600)"=w325, "data bits (8)"=w324, "parity (0:none)"=w326, "error in (no error)"=w319, "flow control (0:none)"=w323) -> ("VISA resource name out"=w320:refnum<visa-resource-name>, "error out"=w318:errorcluster)  [unwired: 6 out]
        n119 = Bundle By Name(cluster=w322, "VISA Resource Name"=w320) -> (w321:T4)
        n120 = call <vilib>:"Add State(s) to Queue__JKI_lib_State_Machine.vi"("State(s) in (\"\")"=w330) -> ("States Out"=w329:string)  [unwired: 14 in]
      }
      frame "Disconnect" {
        # "Do not put any code in this frame.\n(it is a separator no-op)"
        n121 = Unbundle By Name(w332) -> ("VISA Resource Name"=w331:refnum<visa-resource-name>)
        n122 = VISA Flush I/O Buffer(VISA resource name=w331, error in (no error)=w333) -> (VISA resource name out=w336:refnum<visa-resource-name>, error out=w335:errorcluster)  [unwired: 1 in]
        n123 = VISA Close(VISA resource name=w336, error in (no error)=w335) -> (error out=w334:errorcluster)
        n124 = call <vilib>:"Add State(s) to Queue__JKI_lib_State_Machine.vi"("State(s) in (\"\")"=w338) -> ("States Out"=w337:string)  [unwired: 14 in]
      }
      frame "Status" {
        # "Do not put any code in this frame.\n(it is a separator no-op)"
        n125 = Unbundle By Name(w342) -> ("VISA Resource Name"=w354:refnum<visa-resource-name>)
        n126 = Concatenate Strings("STATUS=?" ("string"), "\r" ("string")) -> (w353:string)
        n127 = flat-sequence {
          tunnel: w354 -> [w365]
          tunnel: w353 -> [w364]
          tunnel: w352 -> [w363]
          tunnel: [w362] -> w350
          tunnel: [w361] -> w348
          tunnel: [w367] -> w351
          tunnel: w350 -> [w367]
          tunnel: [w366] -> w349
          tunnel: w348 -> [w366]
          frame #0 {
            n128 = VISA Write(VISA resource name=w365, write buffer=w364, error in (no error)=w363) -> (VISA resource name out=w361:refnum<visa-resource-name>, error out=w362:errorcluster)  [unwired: 1 out]
          }
          frame #1 {
            n129 = Wait (ms)(milliseconds to wait=u32 300) -> ()  [unwired: 1 out]
          }
        }
        n130 = property class="Instr"(reference=w349, error in=w351) -> (reference out=w345:refnum<visa-resource-name>, error out=w343:errorcluster, "Bytes at Port"=w344:u32)
        n131 = VISA Read(VISA resource name=w345, byte count=w344, error in (no error)=w343) -> (read buffer=w347:string, error out=w346:errorcluster)  [unwired: 2 out]
        n132 = call "SplitStatus.vi"("Index"=13, "Input String"=w347) -> ("Out"=w340:string)  [unwired: 9 in]
        "Laser" <- w340
        n133 = call "SplitStatus.vi"("Index"=15, "Input String"=w347) -> ("Out"=w339:string)  [unwired: 9 in]
        "Pump" <- w339
        n134 = Bundle By Name(cluster=w342, "Laser Status"=w340, "Pump Status"=w339) -> (w341:T4)
        n135 = call <vilib>:"Add State(s) to Queue__jki_lib_state_machine.vi"("State(s) in (\"\")"=w360) -> ("States Out"=w359:string)  [unwired: 14 in]
      }
      frame "Write Command" {
        # "Do not put any code in this frame.\n(it is a separator no-op)"
        n136 = Unbundle By Name(w381) -> ("VISA Resource Name"=w380:refnum<visa-resource-name>, "Write Buffer"=w370:string)
        n137 = flat-sequence {
          tunnel: w380 -> [w388]
          tunnel: w379 -> [w387]
          tunnel: [w386] -> w377
          tunnel: [w385] -> w375
          tunnel: w370 -> [w384]
          tunnel: [w390] -> w378
          tunnel: w377 -> [w390]
          tunnel: [w389] -> w376
          tunnel: w375 -> [w389]
          frame #0 {
            n138 = VISA Write(VISA resource name=w388, write buffer=w384, error in (no error)=w387) -> (VISA resource name out=w385:refnum<visa-resource-name>, error out=w386:errorcluster)  [unwired: 1 out]
          }
          frame #1 {
            n139 = Wait (ms)(milliseconds to wait=u32 300) -> ()  [unwired: 1 out]
          }
        }
        n140 = property class="Instr"(reference=w376, error in=w378) -> (reference out=w373:refnum<visa-resource-name>, error out=w371:errorcluster, "Bytes at Port"=w372:u32)
        n141 = VISA Read(VISA resource name=w373, byte count=w372, error in (no error)=w371) -> (error out=w374:errorcluster)  [unwired: 3 out]
        n142 = call <vilib>:"Add State(s) to Queue__JKI_lib_State_Machine.vi"("State(s) in Front (\"\")"="Status\nLog" ("State(s) in Front (\"\")"), "State(s) in (\"\")"=w383) -> ("States Out"=w382:string)  [unwired: 13 in]
      }
      frame "Log" {
        w393 = "\t" ("string")
        # "Set file mark to\nend of file"
        # "Do not put any code in this frame.\n(it is a separator no-op)"
        n143 = Unbundle By Name(w407) -> ("Laser Status"=w394:string, "Write Buffer"=w392:string)
        n144 = Get Date/Time In Seconds() -> (seconds since 1Jan1904=w408:timestamp)
        n145 = Format Date/Time String(time format string (%c)="%Y-%m-%d-%H-%M-%S", seconds (now)=w408) -> (date/time string=w406:string)  [unwired: 1 in]
        n146 = Open/Create/Replace File(file path (use dialog)=path "G:/My Drive/ansom/users/Pubudu/Element2/e2_log.txt" ("file (use dialog)"), error in=w398, operation (0:open)=T3."open or create") -> (refnum out=w402:refnum<file>, error out=w401:errorcluster)  [unwired: 3 in, 1 out]
        n147 = Concatenate Strings(w406, w393, w394, w393, w392) -> (w396:string)
        n148 = Set File Position(offset (in bytes) (0)=i64 0, refnum=w402, from (0:start)=enum16{"start", "end", "current"}."end", error in=w401) -> (refnum out=w404:refnum<file>, error out=w405:errorcluster)
        n149 = Write to Text File(file (use dialog)=w404, text=w396, error in=w405) -> (error out=w397:errorcluster)  [unwired: 1 in, 2 out]
        n150 = call <vilib>:"Add State(s) to Queue__JKI_lib_State_Machine.vi"("State(s) in (\"\")"=w411) -> ("States Out"=w410:string)  [unwired: 14 in]
      }
    }
    "Error" <- w9
  }
